vi "Populate Menu Activation.vi"(8 "error in (no error)":errorcluster, 9 "Coords":T1, 10 "MenuRef":refnum<k9>, 11 "Selector in":refnum<class "Selector.lvclass">) -> (0 "error out":errorcluster, 3 "Selector out":refnum<class "Selector.lvclass">)   [LabVIEW 2019, in "Selector.lvclass"]
uses:
  Selector.lvclass
  <vilib>/Utility/miscctls.llb/LVPoint32TypeDef.ctl
  Selector.lvclass/Selector.ctl
  f1f0a02b-b8b6-4cc5-b4ed-f95812147d19.vi
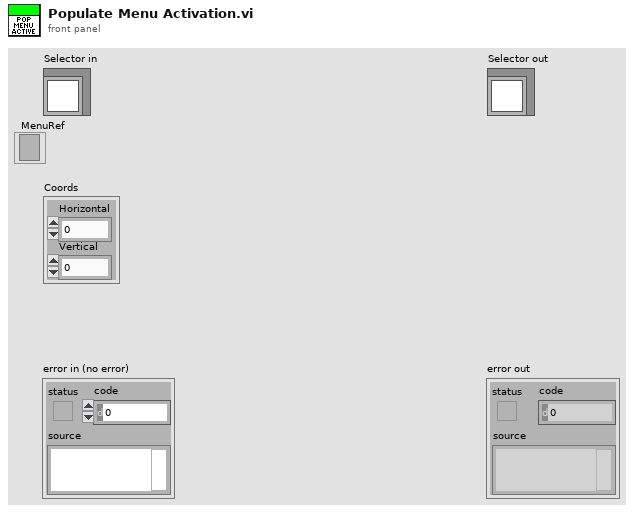
[diagram p1: front panel]
types:
  T1 = typedef "LVPoint32TypeDef.ctl" = cluster{"Horizontal":i32, "Vertical":i32}
  T2 = typedef "LVRowAndColumnTypeDef.ctl" = cluster{"Row":i32, "Column":i32}
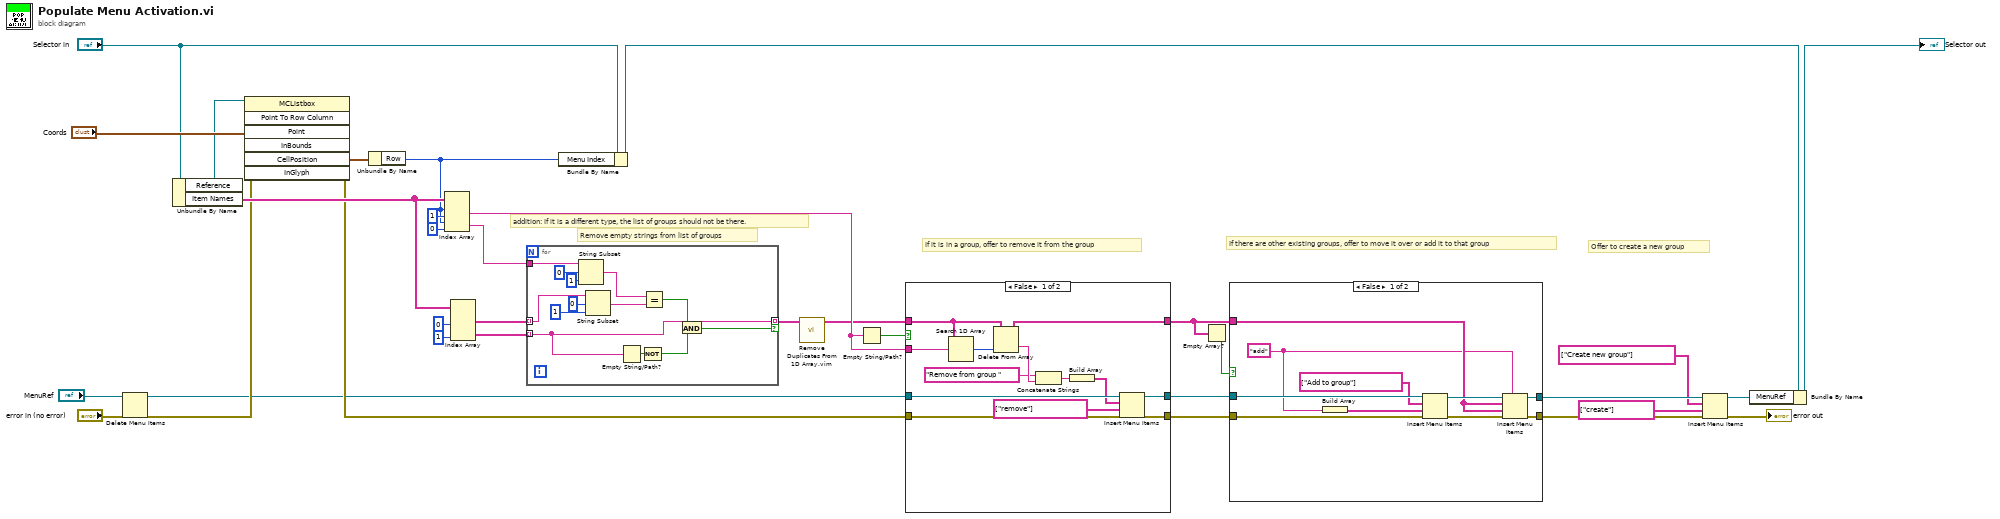
[diagram p0: block diagram]
diagram:
  # "Remove empty strings from list of groups"
  # "addition: If it is a different type, the list of groups should not be there."
  # "Offer to create a new group"
  # "If there are other existing groups, offer to move it over or add it to that group"
  # "If it is in a group, offer to remove it from the group"
  n1 = Delete Menu Items(6:"error in (no error)", 9:"MenuRef") -> (0:w27:errorcluster, 3:w23:refnum<k9>)  [unwired: 2 in]
  n2 = Unbundle By Name("Selector in") -> ("Reference"=w13:refnum<vi>, "Item Names"=w29:string[][])
  n3 = invoke class="MCListbox" method="Point To Row Column"(reference=w13, error in=w27, "Point"="Coords") -> (error out=w24:errorcluster, "CellPosition"=w31:T2)  [unwired: 4 in, 5 out]
  n4 = Unbundle By Name(w31) -> ("Row"=w8:i32)
  n5 = Index Array(array=w29, index (row) #1=w8, index (col) #1=1 ("disabled index (col)"), index (row) #2=w8, index (col) #2=0 ("disabled index (col)")) -> (element #1=w25:string, element #2=w6:string)
  n6 = Index Array(array=w29, index (col) #1=0 ("disabled index (col)"), index (col) #2=1 ("index (col)")) -> (element #1=w2:string[], element #2=w1:string[])  [unwired: 2 in]
  n7 = for {
    tunnel: w6 -> [w47]
    tunnel: [w36] -> w4 mode=indexing if=w35
    tunnel: w2 -> [w38] mode=indexing
    tunnel: w1 -> [w36] mode=indexing
    n8 = String Subset(string=w47, offset (0)=0, length (rest)=1 ("length (rest)")) -> (substring=w41:string)
    n9 = String Subset(string=w38, offset (0)=0, length (rest)=1 ("length (rest)")) -> (substring=w42:string)
    n10 = Empty String/Path?(string/path=w36) -> (empty?=w40:bool)
    n11 = Not(x=w40) -> (.not. x?=w39:bool)
    n12 = Equal?(x=w41, y=w42) -> (x = y?=w37:bool)
    n13 = And(x=w37, y=w39) -> (x .and. y?=w35:bool)
  }
  n14 = Bundle By Name(cluster="Selector in", "Menu Index"=w8) -> (w10:refnum<class "Selector.lvclass">)
  n15 = call "Remove Duplicates From 1D Array.vim"("array"=w4) -> ("array with duplicates removed"=w5:string[])  [unwired: 10 in]
  n16 = Empty String/Path?(string/path=w25) -> (empty?=w26:bool)
  n17 = case shown="False" w26 {
    tunnel: w5 -> [w59 w63]
    tunnel: w25 -> [w60 _]
    tunnel: [w50 w63] -> w19
    tunnel: w24 -> [w53 w61]
    tunnel: [w52 w61] -> w21
    tunnel: w23 -> [w57 w62]
    tunnel: [w51 w62] -> w22
    frame False {
      n18 = Search 1D Array(1D array=w59, element=w60) -> (index of element=w58:i32)  [unwired: 1 in]
      n19 = Delete From Array(array=w59, index=w58) -> (deleted portion=w56:string, array with subset deleted=w50:string[])  [unwired: 1 in]
      n20 = Concatenate Strings("Remove from group " ("string"), w56) -> (w55:string)
      n21 = Build Array(w55) -> (w48:string[])
      n22 = Insert Menu Items(6:w53, 7:string[] ["remove"] ("item tags"), 8:w48, 9:w57) -> (0:w52:errorcluster, 3:w51:refnum<k9>)  [unwired: 2 in, 1 out]
    }
    frame True {
    }
  }
  n23 = Empty Array?(array=w19) -> (empty?=w20:bool)
  n24 = case shown="False" w20 {
    tunnel: w22 -> [w73 w75]
    tunnel: w21 -> [w72 w74]
    tunnel: [w69 w74] -> w16
    tunnel: w19 -> [w68 _]
    tunnel: [w67 w75] -> w18
    frame False {
      w64 = "add" ("menu tag")
      n25 = Build Array(w64) -> (w66:string[])
      n26 = Insert Menu Items(6:w72, 7:w66, 8:string[] ["Add to group"] ("item names"), 9:w73) -> (0:w70:errorcluster, 3:w71:refnum<k9>)  [unwired: 2 in, 1 out]
      n27 = Insert Menu Items(5:w64, 6:w70, 7:w68, 8:w68, 9:w71) -> (0:w69:errorcluster, 3:w67:refnum<k9>)  [unwired: 1 in, 1 out]
    }
    frame True {
    }
  }
  n28 = Insert Menu Items(6:w16, 7:string[] ["create"] ("item tags"), 8:string[] ["Create new group"] ("item names"), 9:w18) -> (0:→"error out":errorcluster, 3:w11:refnum<k9>)  [unwired: 2 in, 1 out]
  n29 = Bundle By Name(cluster=w10, "MenuRef"=w11) -> (→"Selector out":refnum<class "Selector.lvclass">)
